vi "tcs_getSample_kernelTrackingTarget.vi"(8 "error in (no error)":errorcluster, 11 "kernel_TrackingTarget_Ctl":T1) -> (0 "error out":errorcluster, 2 "function return":i32, 3 "kernel_TrackingTarget_Ctl out":T1)   [LabVIEW 2016, in "SALLV_tcs.lvlib"]
doc: "int tcs_shm_getSample_kernel_TrackingTargetLV(tcs_kernel_TrackingTargetLV *kernel_TrackingTarget_Ctl );"
uses:
  SALLV_tcs.lvlib
  DataTypes/kernel_TrackingTarget.ctl
  SALLV_tcs.so
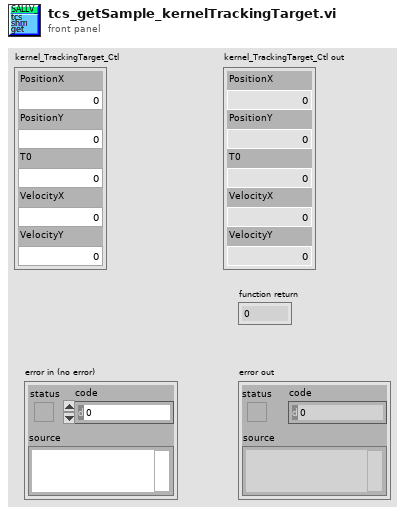
[diagram p1: front panel]
types:
  T1 = typedef "SALLV_tcs.lvlib/kernel_TrackingTarget.ctl" = cluster{"PositionX":sgl, "PositionY":sgl, "T0":sgl, "VelocityX":sgl, "VelocityY":sgl}
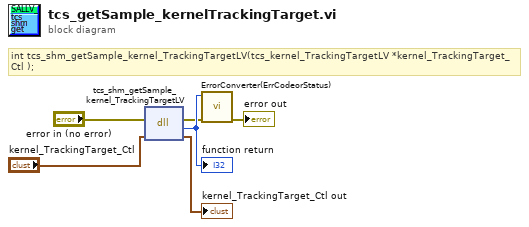
[diagram p0: block diagram]
diagram:
  # "int tcs_shm_getSample_kernel_TrackingTargetLV(tcs_kernel_TrackingTargetLV *kernel_TrackingTarget_Ctl );"
  n1 = dll-call lib="home/andres/Desktop/SALLV_tcs/SALLV_tcs.*" fn="tcs_shm_getSample_kernel_TrackingTargetLV"(error in="error in (no error)", "kernel_TrackingTarget_Ctl"="kernel_TrackingTarget_Ctl") -> (error out=w2:errorcluster, w6:i32, "kernel_TrackingTarget_Ctl"=→"kernel_TrackingTarget_Ctl out":T1)  [unwired: 2 in, 1 out]
  "function return" <- w6
  n2 = call "ErrorConverter(ErrCodeorStatus).vi"("error in (no error)"=w2, "error code"=w6) -> ("error out"=→"error out":errorcluster)  [unwired: 9 in]
